vi "Read Name of Device.vi"(8 "error in (no error)":errorcluster, 11 "DAQdevice in":refnum<class "DAQdevice.lvclass">) -> (0 "error out":errorcluster, 2 "Name of Device":string, 3 "DAQdevice out":refnum<class "DAQdevice.lvclass">)   [LabVIEW 2016, in "DAQdevice.lvclass"]
uses:
  DAQdevice.lvclass
  DAQdevice.lvclass/DAQdevice.ctl
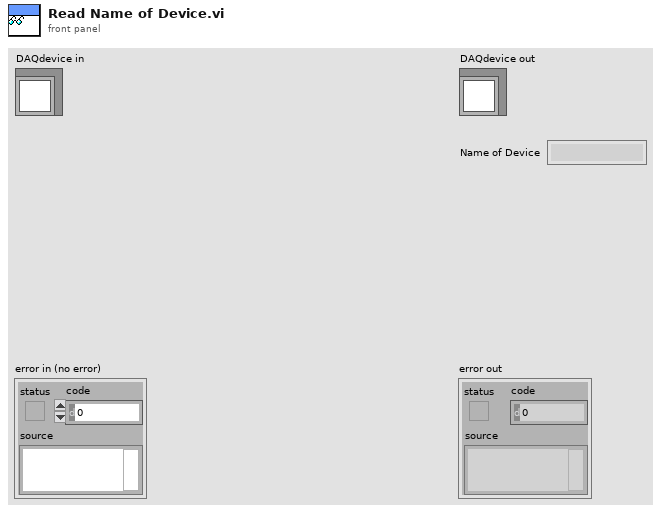
[diagram p1: front panel]
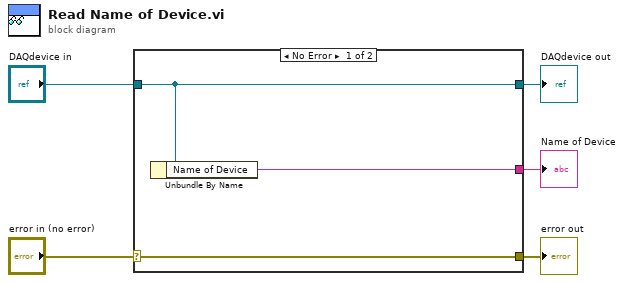
[diagram p0: block diagram]
diagram:
  n1 = case shown="No Error" "error in (no error)" {
    selector: "error in (no error)" -> [w8 w9]
    tunnel: [w8 w9] -> w4
    tunnel: [w7 w10] -> w2
    tunnel: "DAQdevice in" -> [w7 w10]
    tunnel: [w6 _] -> w1
    frame No Error {
      n2 = Unbundle By Name(w7) -> ("Name of Device"=w6:string)
    }
    frame Error {
    }
  }
  "error out" <- w4
  "DAQdevice out" <- w2
  "Name of Device" <- w1
